vi "Move_Arm_to_Camera.vi"(0 "VISA Refnum in":refnum<visa-resource-name>="COM3", 1 "error in":errorcluster) -> (7 "Machine Out":refnum<visa-resource-name>, 8 "error out":errorcluster)   [LabVIEW 2018]
doc: "Example interface for controlling uArm Swift Pro."
panel:
  in  "Write Buffer":string="G90 G0 X1\n"
  out "read buffer":string
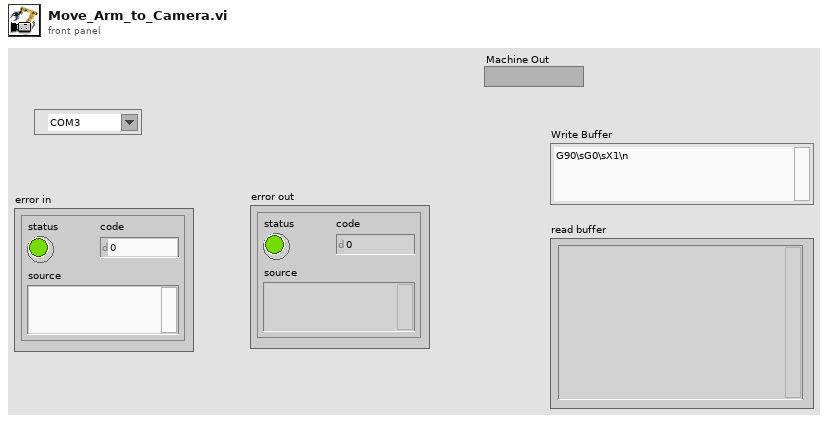
[diagram p1: front panel]
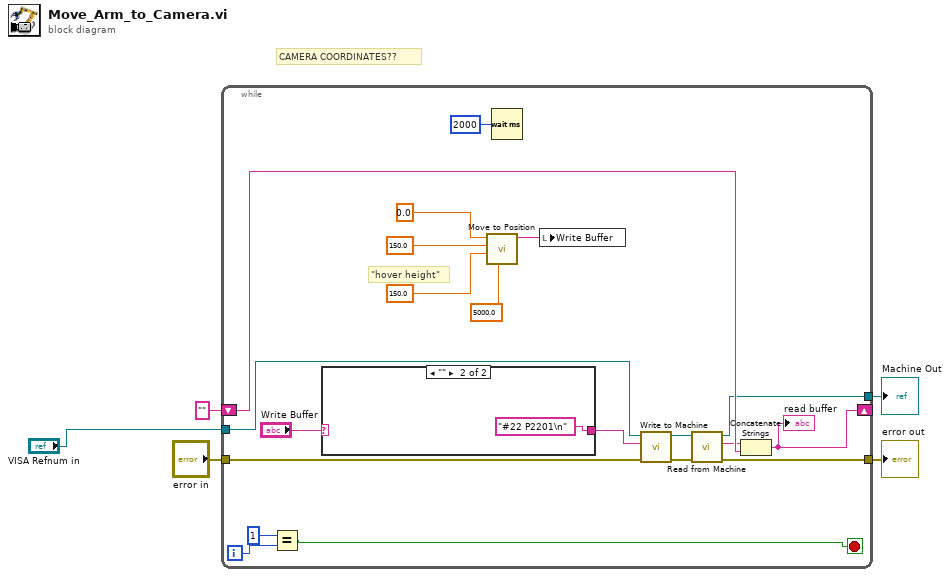
[diagram p0: block diagram]
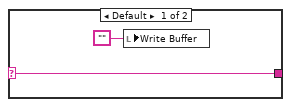
[diagram p2: hidden frame]
diagram:
  # "CAMERA COORDINATES??"
  n1 = while {
    tunnel: "VISA Refnum in" -> [w23]
    tunnel: "error in" -> [w20]
    shift-right: [w21] -> _
    shift-left: "" -> [w22]
    tunnel: [w19] -> w1
    tunnel: [w15] -> w2
    i -> [w10]
    stop <- w8 stop-if-true
    # "\"hover height\""
    n2 = Equal?(x=1, y=w10) -> (x = y?=w8:bool)
    n3 = case shown="\"\"" "Write Buffer" {
      selector: "Write Buffer" -> [w27 _]
      tunnel: [w27 "#22 P2201\n"] -> w24
      frame Default {
        n4 = local write "Write Buffer"("") -> ()
      }
      frame "" {
      }
    }
    n5 = call "Move to Position.vi"("Speed"=5000.0, "Z-Position"=150.0, "Y-Position"=150.0 ("X-position"), "X-Position"=0.0 ("Y-position")) -> ("G-Code String"=w12:string)  [unwired: 7 in]
    n6 = Wait (ms)(milliseconds to wait=u32 2000) -> ()  [unwired: 1 out]
    n7 = local write "Write Buffer"(w12) -> ()
    n8 = call "Write to Machine .vi"("error in (no error)"=w20, "G-Code String In"=w24, "Machine In"=w23) -> ("error out"=w17:errorcluster, "Machine Out"=w16:refnum<visa-resource-name>)  [unwired: 7 in]
    n9 = call "Read from Machine.vi"("error in (no error)"=w17, "Machine In"=w16) -> ("error out"=w15:errorcluster, "read buffer"=w18:string, "Machine Out"=w19:refnum<visa-resource-name>)  [unwired: 7 in]
    n10 = Concatenate Strings(w18, w22) -> (w21:string)
    "read buffer" <- w21
  }
  "error out" <- w2
  "Machine Out" <- w1
